vi "stringToXML.vi"(8 "error in (no error)":errorcluster, 10 "xmlString":string) -> (0 "error out":errorcluster, 3 "NativeXML out":refnum<class "NativeXML.lvclass">)   [LabVIEW 2011, in "Tools.lvlib" / "xml.lvlib" / "NativeXML.lvclass"]
uses:
  NativeXML.lvclass
  NativeXML.lvclass/NativeXML.ctl
  <vilib>/xml/Load XML String.vi
  <vilib>/xml/NI_XML.lvlib
  Program Files/National Instruments/LabVIEW 2011/resource/objmgr/DOMUserDefRef.rc
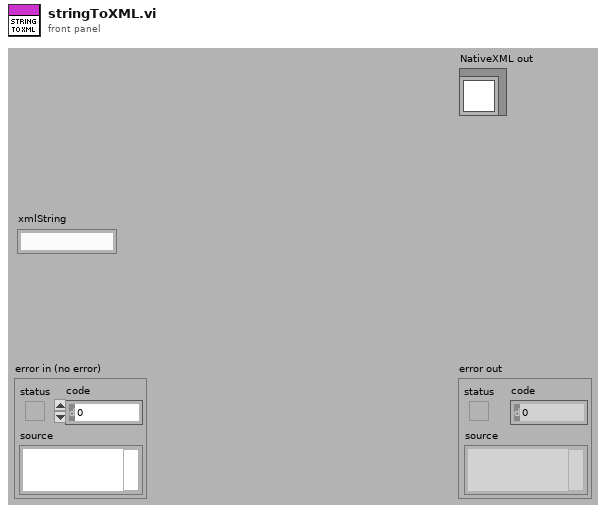
[diagram p1: front panel]
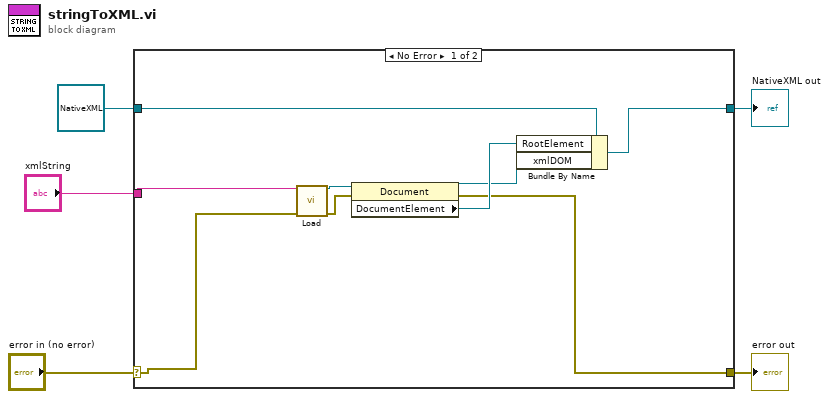
[diagram p0: block diagram]
diagram:
  n1 = case shown="No Error" "error in (no error)" {
    selector: "error in (no error)" -> [w7 w16]
    tunnel: [w8 w16] -> w4
    tunnel: [w10 w15] -> w3
    tunnel: refnum<class "NativeXML.lvclass"> refnum ("Tools.lvlib:xml.lvlib:NativeXML.lvclass") -> [w11 w15]
    tunnel: "xmlString" -> [w14 _]
    frame No Error {
      n2 = call-poly <vilib>:"Load.vi"("XML string"=w14, "error in (no error)"=w7) -> ("DOM document out"=w13:refnum<k20>, "error out"=w12:errorcluster)  [unwired: 11 in, 1 out]
      n3 = property class="Document"(reference=w13, error in=w12) -> (reference out=w6:refnum<k20>, error out=w8:errorcluster, "DocumentElement"=w9:refnum<k20>)
      n4 = Bundle By Name(cluster=w11, "RootElement"=w9, "xmlDOM"=w6) -> (w10:refnum<class "NativeXML.lvclass">)
    }
    frame Error {
    }
  }
  "error out" <- w4
  "NativeXML out" <- w3
